vi "GetCustomData.vi"(8 "error in":errorcluster, 11 "Document in":refnum<class "Document.lvclass">) -> (0 "error out":errorcluster, 2 "CustomData":refnum<class "CustomData.lvclass">, 3 "Document out":refnum<class "Document.lvclass">)   [LabVIEW 2021, in "ProligentXMLGenerator.lvlib" / "Document.lvclass"]
doc: "Get CustomElement."
uses:
  Document.lvclass
  Document.lvclass/Document.ctl
  CustomData/CustomData.lvclass
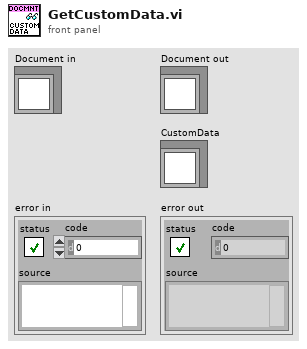
[diagram p1: front panel]
types:
  T1 = typedef "ProligentXMLGenerator.lvlib/Document.lvclass/Data.ctl" = cluster{"Name":string, "CustomData":refnum<class "CustomData.lvclass">, "Identifier":refnum<class "Guid.lvclass">, "NameType":refnum<class "NonEmptyString_255.lvclass">, "FileName":refnum<class "NonEmptyString_255.lvclass">, "Description":refnum<class "NonNullableString_600.lvclass">, "FilePath":path, "DestinationFolder":path}
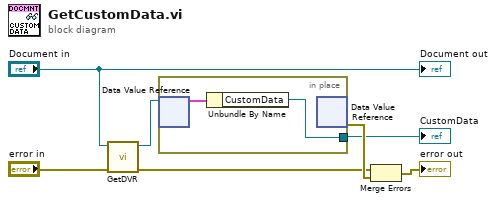
[diagram p0: block diagram]
diagram:
  n1 = call "GetDVR.vi"("error in"="error in", "Document in"="Document in") -> ("error out"=w2:errorcluster, "DVRReference"=w6:refnum<data-value>)  [unwired: 8 in]
  n2 = in-place "In Place Element Structure" {
    in-place-border: [w8] -> w1
    n3 = in-place-dvr #1(w6) -> (w9:T1)  [unwired: 1 out]
    n4 = Unbundle By Name(w9) -> ("CustomData"=w8:refnum<class "CustomData.lvclass">)
    n5 = in-place-dvr #1() -> (w7:errorcluster)  [unwired: 1 in, 1 out]
  }
  "CustomData" <- w1
  n6 = Merge Errors(w2, w7) -> (→"error out":errorcluster)
  "Document out" <- "Document in"
